vi "TestFGVBedVacant.vi"() -> (0 "error out":errorcluster, 2 "Pass":bool)   [LabVIEW 2015]
uses:
  LVClasses/Flags/ColorFlags.ctl
  TypeDef/RoomsActionEnum.ctl
  LVClasses/Flags/Flags.lvclass
panel:
  out "Data Out 2":string
  out "Data Out":string
  in  "State":bool[](array[boolean])=[FALSE, FALSE, FALSE, FALSE]
  out "Flags Read 1":T1={"Flag State"=[1, 3, 5, 7]}
  out "Flags Write":T1={"Flag State"=[1, 3, 5, 7]}
  out "Flags Read 2":T1={"Flag State"=[1, 3, 5, 7]}
  in  "FGV Room":i32=102
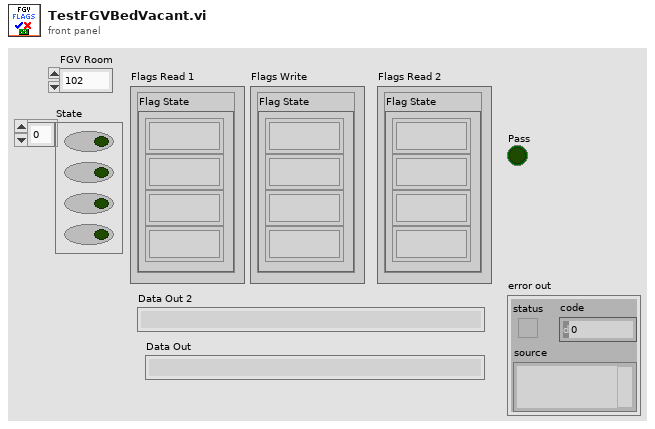
[diagram p1: front panel]
types:
  T1 = typedef "Flags.lvclass/ColorFlags.ctl" = cluster{"Flag State":u8[]}
  T2 = typedef "RoomsActionEnum.ctl" = enum16{"Init", "Add Room", "Remove Room", "Read Room", "Read Flag", "Read Flag State", "Write Flag State", "Read Flag Color", "Write Flag Color", "Read Bed Vacant", "Write Bed Vacant", "Read Personnel", "Add Personnel", "Remove Personnel", "Read Requests", "Add Request", "Remove Request", "Read Beacon ID", "Write Beacon ID", "Write Bed URL", "Read Bed URL"}
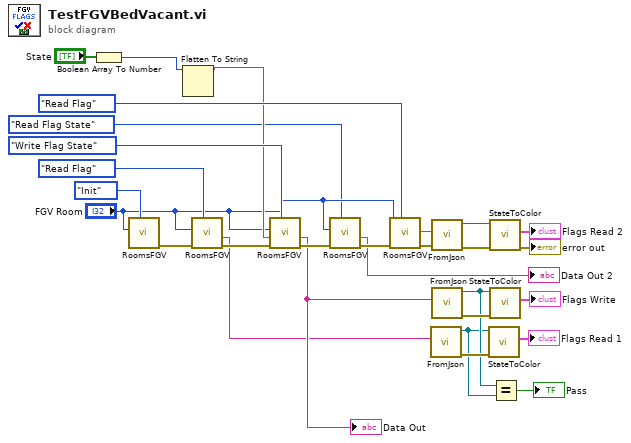
[diagram p0: block diagram]
diagram:
  n1 = Boolean Array To Number(Boolean array="State") -> (number=w5:u32)
  n2 = call "RoomsFGV.vi"("Actions"=RoomsActionEnum."Init", "Room"="FGV Room") -> ("error out"=w28:errorcluster)  [unwired: 8 in, 1 out]
  n3 = Flatten To String(anything=w5) -> (data string=w6:string)  [unwired: 3 in, 2 out]
  n4 = call "RoomsFGV.vi"("Actions"=RoomsActionEnum."Read Flag", "error in (no error)"=w28, "Room"="FGV Room") -> ("error out"=w27:errorcluster, "Data Out"=w13:string)  [unwired: 7 in]
  n5 = call "RoomsFGV.vi"("Actions"=RoomsActionEnum."Write Flag State", "error in (no error)"=w27, "Data In"=w6, "Room"="FGV Room") -> ("error out"=w26:errorcluster, "Data Out"=w14:string)  [unwired: 6 in]
  "Data Out" <- w14
  n6 = call "RoomsFGV.vi"("Actions"=RoomsActionEnum."Read Flag State", "error in (no error)"=w26, "Room"="FGV Room") -> ("error out"=w4:errorcluster, "Data Out"=→"Data Out 2":string)  [unwired: 7 in]
  n7 = call "RoomsFGV.vi"("Actions"=RoomsActionEnum."Read Flag", "error in (no error)"=w4, "Room"="FGV Room") -> ("error out"=w23:errorcluster, "Data Out"=w15:string)  [unwired: 7 in]
  n8 = call "FromJson.vi"("String"=w13) -> ("error out"=w17:errorcluster, "Flags out"=w11:refnum<class "Flags.lvclass">)  [unwired: 9 in]
  n9 = call "FromJson.vi"("error in (no error)"=w23, "String"=w15) -> ("error out"=w21:errorcluster, "Flags out"=w22:refnum<class "Flags.lvclass">)  [unwired: 8 in]
  n10 = call "FromJson.vi"("String"=w14) -> ("error out"=w18:errorcluster, "Flags out"=w12:refnum<class "Flags.lvclass">)  [unwired: 9 in]
  n11 = call "StateToColor.vi"("error in (no error)"=w17, "Flags in"=w11) -> ("RoomNumFlags"=→"Flags Read 1":T1)  [unwired: 7 in, 2 out]
  n12 = call "StateToColor.vi"("error in (no error)"=w21, "Flags in"=w22) -> ("error out"=→"error out":errorcluster, "RoomNumFlags"=→"Flags Read 2":T1)  [unwired: 7 in, 1 out]
  n13 = call "StateToColor.vi"("error in (no error)"=w18, "Flags in"=w12) -> ("RoomNumFlags"=→"Flags Write":T1)  [unwired: 7 in, 2 out]
  n14 = Equal?(x=w12, y=w11) -> (x = y?=→"Pass":bool)
